vi "Set Shared Variable Refnum.vi"(8 "error in (no error)":errorcluster, 10 "shared variable refnum":refnum<k21>, 11 "abs_SharedVariable in":refnum<class "abs_SharedVariable.lvclass">) -> (0 "error out":errorcluster, 3 "abs_SharedVariable out":refnum<class "abs_SharedVariable.lvclass">)   [LabVIEW 2021, in "abs_SharedVariable.lvclass"]
doc: "LVabs_Shared Variable 1.0.0.2\nTim - TSA\nCopyright (c) 2024, TSA"
uses:
  abs_SharedVariable.lvclass
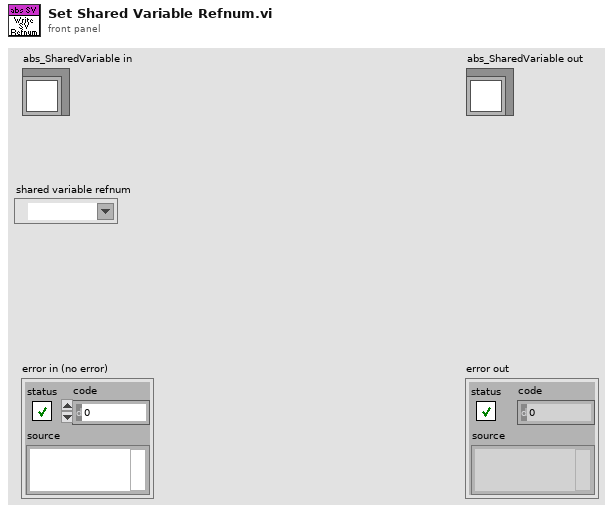
[diagram p1: front panel]
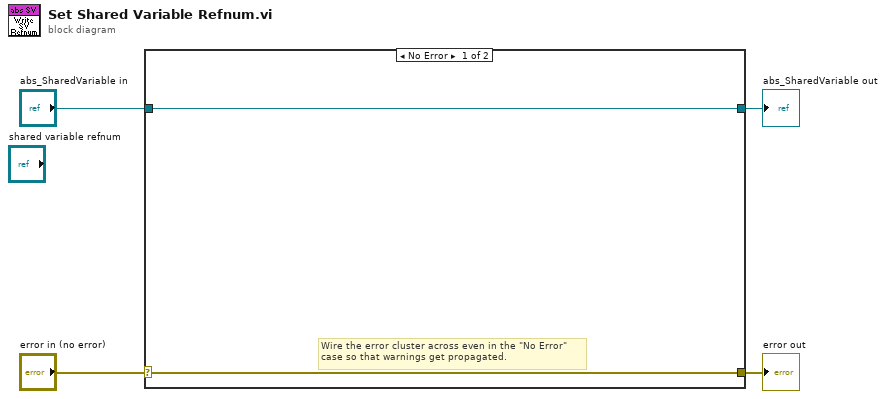
[diagram p0: block diagram]
diagram:
  n1 = case shown="No Error" "error in (no error)" {
    selector: "error in (no error)" -> [w6 w8]
    tunnel: [w6 w8] -> w3
    tunnel: [w5 w7] -> w1
    tunnel: "abs_SharedVariable in" -> [w5 w7]
    frame No Error {
      # "Wire the error cluster across even in the \"No Error\"\ncase so that warnings get propagated."
    }
    frame Error {
    }
  }
  "error out" <- w3
  "abs_SharedVariable out" <- w1
